vi "Main Settings FG.vi"(6 "Action":enum8{"GET", "SET"}(ring), 8 "error in (no error)":errorcluster, 10 "Main Settings":T1={"RIO Device Address"="RIO0", "Local bitfile path"=path "", "RT bitfile path"=path "", "Number of injectors"=0, "Max injection shot count"=1, "Sample rate (S/s)"=500000, "Stages"=["Boost", "Battery", "Off"]}, 11 "Item Ref":T2 format="%.0x") -> (0 "error out":errorcluster, 2 "Main Settings out":T1, 3 "Item Ref out":T2=18446744073709551615 format="%.0x")   [LabVIEW 2015, in "Fuel Injection Addon Shared.lvlib"]
uses:
  Fuel Injection Addon Shared.lvlib
  <vilib>/NI Veristand/Custom Device API/Custom Device Item Ref.ctl
  Types/Main Settings.ctl
  Constants.vi
  <vilib>/NI Veristand/Custom Device API/Get Item Property (Path).vi
  <vilib>/NI Veristand/Custom Device API/Get Item Property (U16).vi
  <vilib>/NI Veristand/Custom Device API/Get Item Property (String).vi
  <vilib>/NI Veristand/Custom Device API/Get Item Property (U32).vi
  <vilib>/NI Veristand/Custom Device API/Get Item Property (Variant).vi
  <vilib>/NI Veristand/Custom Device API/Set Item Property (Path).vi
  <vilib>/NI Veristand/Custom Device API/Set Item Property (String).vi
  <vilib>/NI Veristand/Custom Device API/Set Item Property (U16).vi
  <vilib>/NI Veristand/Custom Device API/Set Item Property (U32).vi
  <vilib>/NI Veristand/Custom Device API/Set Item Property (Variant).vi
  <vilib>/NI VeriStand/Custom Device API/Custom Device API.lvlib
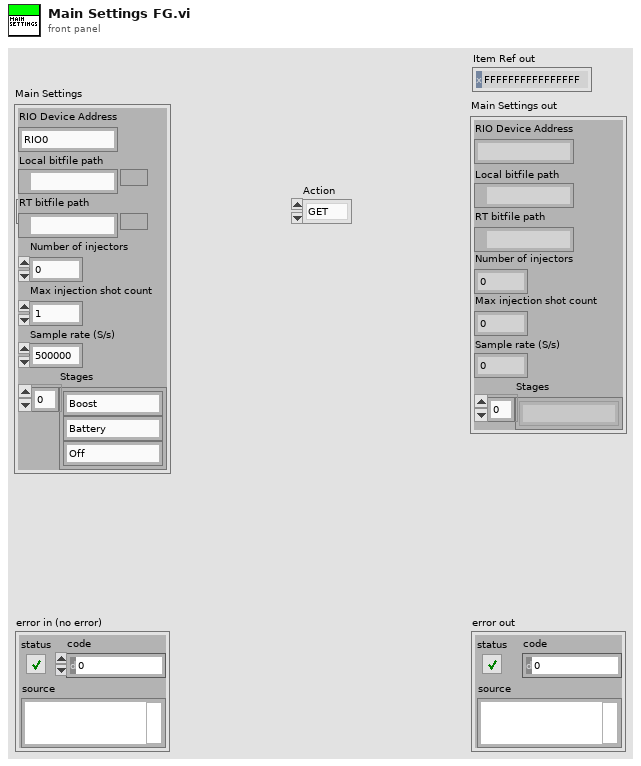
[diagram p1: front panel]
types:
  T1 = typedef "Fuel Injection Addon Shared.lvlib/Main Settings.ctl" = cluster{"RIO Device Address":string, "Local bitfile path":path, "RT bitfile path":path, "Number of injectors":u16, "Max injection shot count":u16, "Sample rate (S/s)":u32, "Stages":string[]}
  T2 = typedef "Custom Device API.lvlib/Custom Device Item Ref.ctl" = u64
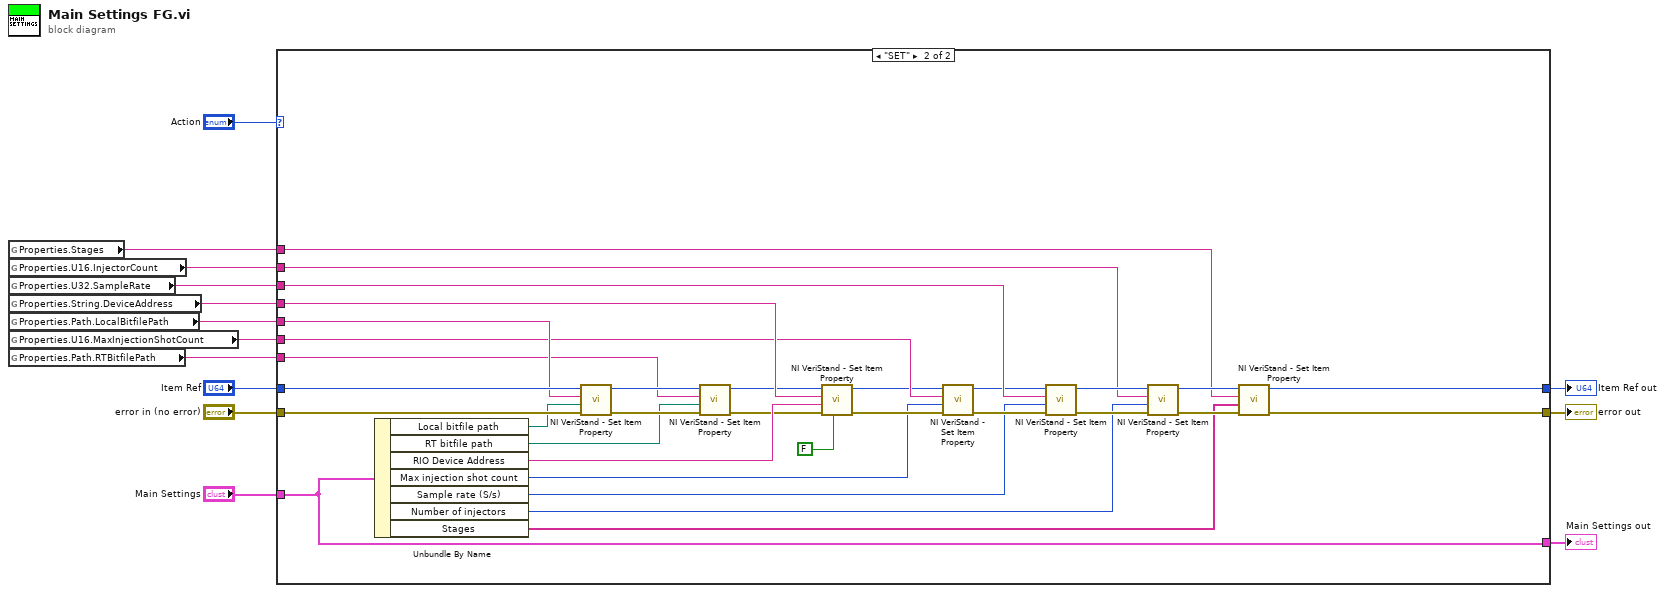
[diagram p0: block diagram]
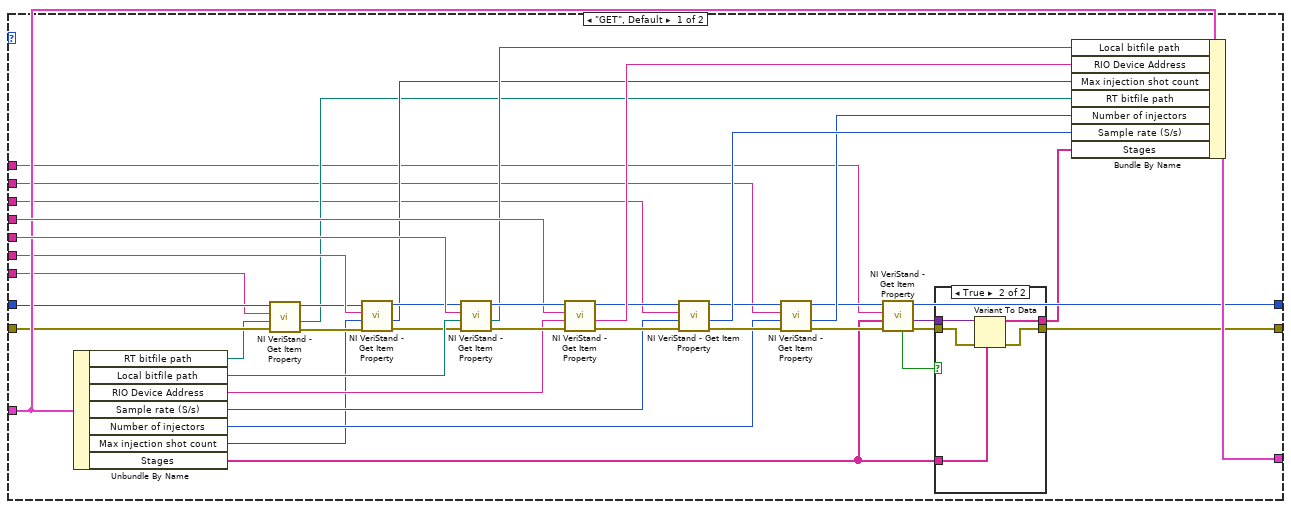
[diagram p2: hidden frame]
diagram:
  n1 = global read "Constants.vi" "Properties.Stages"() -> (w1:string)
  n2 = global read "Constants.vi" "Properties.U16.InjectorCount"() -> (w3:string)
  n3 = global read "Constants.vi" "Properties.U32.SampleRate"() -> (w4:string)
  n4 = global read "Constants.vi" "Properties.String.DeviceAddress"() -> (w8:string)
  n5 = global read "Constants.vi" "Properties.Path.LocalBitfilePath"() -> (w7:string)
  n6 = global read "Constants.vi" "Properties.U16.MaxInjectionShotCount"() -> (w6:string)
  n7 = global read "Constants.vi" "Properties.Path.RTBitfilePath"() -> (w5:string)
  n8 = case shown="\"SET\"" "Action" {
    tunnel: "error in (no error)" -> [w39 w95]
    tunnel: "Item Ref" -> [w40 w94]
    tunnel: "Main Settings" -> [w50 w92]
    tunnel: [w19 w66] -> w10
    tunnel: [w23 w67] -> w13
    tunnel: [w49 w92] -> w2
    tunnel: w7 -> [w56 w93]
    tunnel: w8 -> [w51 w89]
    tunnel: w6 -> [w44 w87]
    tunnel: w5 -> [w38 w82]
    tunnel: w4 -> [w32 w78]
    tunnel: w3 -> [w26 w72]
    tunnel: w1 -> [w15 w64]
    frame "GET", Default {
      n9 = Unbundle By Name(w50) -> ("RT bitfile path"=w36:path, "Local bitfile path"=w53:path, "RIO Device Address"=w52:string, "Sample rate (S/s)"=w33:u32, "Number of injectors"=w28:u16, "Max injection shot count"=w27:u16, "Stages"=w18:string[])
      n10 = call-poly <vilib>:"NI VeriStand - Get Item Property.vi"("error in (no error)"=w39, "Default Value"=w36, "Property Name"=w38, "Item Ref in"=w40) -> ("error out"=w41:errorcluster, "Value"=w37:path, "Item Ref out"=w42:T2)  [unwired: 4 in, 1 out]
      n11 = call-poly <vilib>:"NI VeriStand - Get Item Property.vi"("error in (no error)"=w41, "Default Value"=w27, "Property Name"=w44, "Item Ref in"=w42) -> ("error out"=w45:errorcluster, "Value"=w43:u16, "Item Ref out"=w46:T2)  [unwired: 4 in, 1 out]
      n12 = call-poly <vilib>:"NI VeriStand - Get Item Property.vi"("error in (no error)"=w45, "Default Value"=w53, "Property Name"=w56, "Item Ref in"=w46) -> ("error out"=w54:errorcluster, "Value"=w48:path, "Item Ref out"=w55:T2)  [unwired: 4 in, 1 out]
      n13 = call-poly <vilib>:"NI VeriStand - Get Item Property.vi"("error in (no error)"=w54, "Default Value"=w52, "Property Name"=w51, "Item Ref in"=w55) -> ("error out"=w35:errorcluster, "Value"=w47:string, "Item Ref out"=w34:T2)  [unwired: 4 in, 1 out]
      n14 = call-poly <vilib>:"NI VeriStand - Get Item Property.vi"("error in (no error)"=w35, "Default Value"=w33, "Property Name"=w32, "Item Ref in"=w34) -> ("error out"=w30:errorcluster, "Value"=w31:u32, "Item Ref out"=w29:T2)  [unwired: 4 in, 1 out]
      n15 = call-poly <vilib>:"NI VeriStand - Get Item Property.vi"("error in (no error)"=w30, "Default Value"=w28, "Property Name"=w26, "Item Ref in"=w29) -> ("error out"=w22:errorcluster, "Value"=w25:u16, "Item Ref out"=w24:T2)  [unwired: 4 in, 1 out]
      n16 = call-poly <vilib>:"NI VeriStand - Get Item Property.vi"("error in (no error)"=w22, "Default Value"=w18, "Property Name"=w15, "Item Ref in"=w24) -> ("error out"=w20:errorcluster, "Value"=w21:variant, "Item Ref out"=w23:T2, "Found?"=w17:bool)  [unwired: 4 in]
      n17 = case shown="True" w17 {
        tunnel: w21 -> [_ w63]
        tunnel: w20 -> [w57 w62]
        tunnel: [w57 w61] -> w19
        tunnel: w18 -> [w58 w60]
        tunnel: [w58 w59] -> w16
        frame False {
        }
        frame True {
          n18 = Variant To Data(error in=w62, type=w60, Variant=w63) -> (data=w59:string[], error out=w61:errorcluster)
        }
      }
      n19 = Bundle By Name(cluster=w50, "Local bitfile path"=w48, "RIO Device Address"=w47, "Max injection shot count"=w43, "RT bitfile path"=w37, "Number of injectors"=w25, "Sample rate (S/s)"=w31, "Stages"=w16) -> (w49:T1)
    }
    frame "SET" {
      n20 = Unbundle By Name(w92) -> ("Local bitfile path"=w83:path, "RT bitfile path"=w81:path, "RIO Device Address"=w90:string, "Max injection shot count"=w86:u16, "Sample rate (S/s)"=w73:u32, "Number of injectors"=w71:u16, "Stages"=w65:string[])
      n21 = call-poly <vilib>:"NI VeriStand - Set Item Property.vi"("error in (no error)"=w95, "Value"=w83, "Property Name"=w93, "Item Ref in"=w94) -> ("error out"=w84:errorcluster, "Item Ref out"=w85:T2)  [unwired: 5 in, 1 out]
      n22 = call-poly <vilib>:"NI VeriStand - Set Item Property.vi"("error in (no error)"=w84, "Value"=w81, "Property Name"=w82, "Item Ref in"=w85) -> ("error out"=w80:errorcluster, "Item Ref out"=w79:T2)  [unwired: 5 in, 1 out]
      n23 = call-poly <vilib>:"NI VeriStand - Set Item Property.vi"("Binary String (T)"=FALSE, "error in (no error)"=w80, "Value"=w90, "Property Name"=w89, "Item Ref in"=w79) -> ("error out"=w88:errorcluster, "Item Ref out"=w70:T2)  [unwired: 4 in, 1 out]
      n24 = call-poly <vilib>:"NI VeriStand - Set Item Property.vi"("error in (no error)"=w88, "Value"=w86, "Property Name"=w87, "Item Ref in"=w70) -> ("error out"=w75:errorcluster, "Item Ref out"=w77:T2)  [unwired: 5 in, 1 out]
      n25 = call-poly <vilib>:"NI VeriStand - Set Item Property.vi"("error in (no error)"=w75, "Value"=w73, "Property Name"=w78, "Item Ref in"=w77) -> ("error out"=w74:errorcluster, "Item Ref out"=w76:T2)  [unwired: 5 in, 1 out]
      n26 = call-poly <vilib>:"NI VeriStand - Set Item Property.vi"("error in (no error)"=w74, "Value"=w71, "Property Name"=w72, "Item Ref in"=w76) -> ("error out"=w68:errorcluster, "Item Ref out"=w69:T2)  [unwired: 5 in, 1 out]
      n27 = call-poly <vilib>:"NI VeriStand - Set Item Property.vi"("error in (no error)"=w68, "Value"=w65, "Property Name"=w64, "Item Ref in"=w69) -> ("error out"=w66:errorcluster, "Item Ref out"=w67:T2)  [unwired: 5 in, 1 out]
    }
  }
  "error out" <- w10
  "Item Ref out" <- w13
  "Main Settings out" <- w2
